vi "RunInference.vi"(4 "Introspection Output":T1, 6 "outputIndex":i32, 8 "error in (no error)":errorcluster, 9 "inputIndex":i32, 10 "inputBuffer":sgl[](array[numeric]), 11 "session id in":i32) -> (0 "error out":errorcluster, 1 "Dims":i64[](array[numeric]), 2 "outputBuffer":sgl[](array[numeric]), 3 "session id out":i32, 5 "RunInference":bool)   [LabVIEW 2017, in "libonnx_wrapper.lvlib"]
doc: "/**\n * @brief Выполнить инференс (предсказание) модели\n * \n * Основная функция для получения предсказания от модели. Принимает входные данные,\n * передаёт их в нейросеть и записывает результат в выходной буфер.\n * \n * @param sessionId [IN] ID сессии\n * @param inputIndex [IN] Индекс входа (обычно 0 для моделей с одним входом)\n * @param inputBuffer [IN] Массив входных данных (тип должен соответствовать GetInputType)\n * @param inputSize [IN] Количество элементов во входном массиве\n * @param outputIndex [IN] Индекс выхода (обычно 0 для моделей с одним выходом)\n * @param outputBuffer [OUT] Массив для записи результатов (должен быть выделен в LabVIEW)\n * @param outputSize [IN] Размер выходного буфера в элементах\n * \n * @return int32: 0 при успешном выполнении инференса\n * @return int32: -1 при ошибке (сессия не загружена, неверные индексы, ошибка ONNX Runtime)\n * \n * @note Входные данные должны быть нормализованы так же, как при обучении модели\n * @note Размер входного массива должен соответствовать произведению всех размерностей shape\n * @note Выходной буфер должен быть достаточного размера (см. GetOutputShapeDim)\n * @note Функция блокирует выполнение до завершения инференса\n * \n * @example\n * // Для модели с входом [1, 10] и выходом [1, 3]:\n * float inputData[10] = {...};\n * float outputData[3];\n * RunInference(sessionId, 0, inputData, 10, 0, outputData, 3);\n */\nint RunInference(int sessionId, int inputIndex, float* inputBuffer, int inputSize, \n int outputIndex, float* outputBuffer, int outputSize);"
uses:
  libonnx_wrapper.lvlib
  TypeDef/IO.ctl
  TypeDef/Introspection.ctl
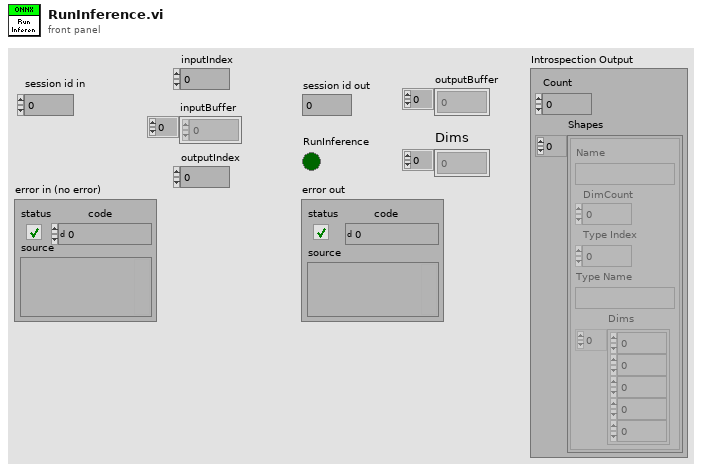
[diagram p1: front panel]
types:
  T1 = typedef "libonnx_wrapper.lvlib/Introspection.ctl" = cluster{"Count":i32, "Shapes":T2[]}
  T2 = typedef "libonnx_wrapper.lvlib/IO.ctl" = cluster{"Name":string, "DimCount":i32, "Type Index":i32, "Type Name":string, "Dims":i64[]}
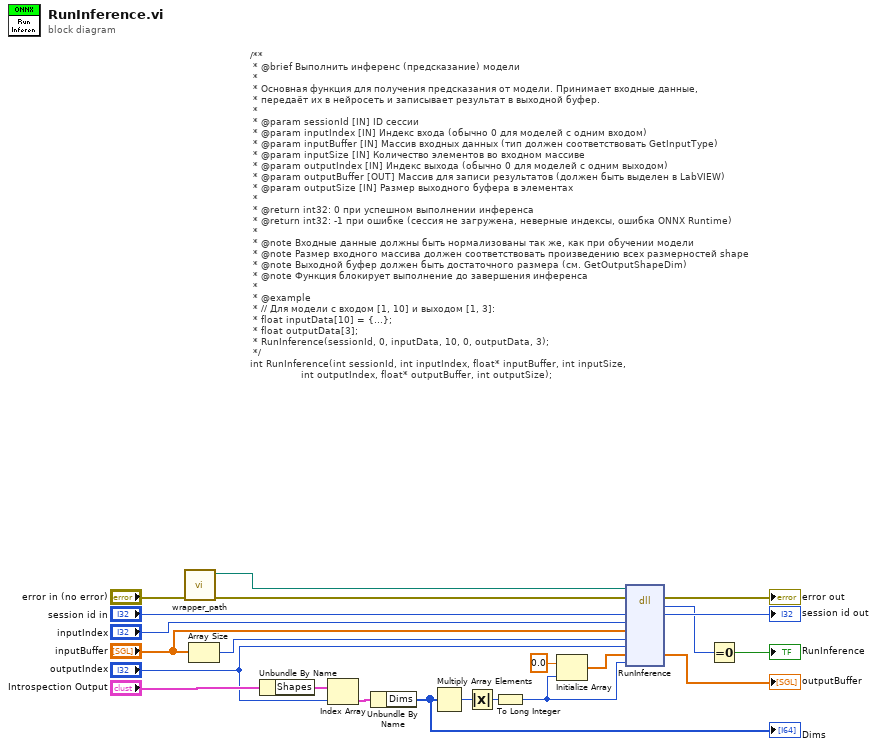
[diagram p0: block diagram]
diagram:
  # "/**\n * @brief Выполнить инференс (предсказание) модели\n * \n * Основная функция для получения предсказания от модели. Принимает входные данные,\n * передаёт их в нейросеть и записывает результат в выходной буфер.\n * \n * @param sessionId [IN] ID сессии\n * @param inputIndex [IN] Индекс входа (обычно 0 для моделей с одним входом)\n * @param inputBuffer [IN] Массив входных данных (тип должен соответствовать GetInputType)\n * @param inputSize [IN] Количество элементов во входном массиве\n * @param outputIndex [IN] Индекс выхода (обычно 0 для моделей с одним выходом)\n * @param outputBuffer [OUT] Массив для записи результатов (должен быть выделен в LabVIEW)\n * @param outputSize [IN] Размер выходного буфера в элементах\n * \n * @return int32: 0 при успешном выполнении инференса\n * @return int32: -1 при ошибке (сессия не загружена, неверные индексы, ошибка ONNX Runtime)\n * \n * @note Входные данные должны быть нормализованы так же, как при обучении модели\n * @note Размер входного массива должен соответствовать произведению всех размерностей shape\n * @note Выходной буфер должен быть достаточного размера (см. GetOutputShapeDim)\n * @note Функция блокирует выполнение до завершения инференса\n * \n * @example\n * // Для модели с входом [1, 10] и выходом [1, 3]:\n * float inputData[10] = {...};\n * float outputData[3];\n * RunInference(sessionId, 0, inputData, 10, 0, outputData, 3);\n */\nint RunInference(int sessionId, int inputIndex, float* inputBuffer, int inputSize, \n                 int outputIndex, float* outputBuffer, int outputSize);"
  n1 = call "wrapper_path.vi"("error in (no error)"="error in (no error)") -> ("error out"=w19:errorcluster, "wrapper path"=w20:path)  [unwired: 9 in]
  n2 = Array Size(array="inputBuffer") -> (size(s)=w12:i32)
  n3 = Unbundle By Name("Introspection Output") -> ("Shapes"=w8:T2[])
  n4 = Index Array(array=w8, index="outputIndex") -> (element=w7:T2)
  n5 = Unbundle By Name(w7) -> ("Dims"=w6:i64[])
  "Dims" <- w6
  n6 = Multiply Array Elements(1:w6) -> (0:w5:i64)
  n7 = Absolute Value(x=w5) -> (abs(x)=w4:i64)
  n8 = To Long Integer(number=w4) -> (32bit integer=w3:i32)
  n9 = Initialize Array(sgl 0.0 ("element"), w3) -> (w10:sgl[])
  n10 = dll-call lib="home/ivan/LabVIEWData/ONNX/Test/libonnx_wrapper/unix64/libonnx_wrapper.*" fn="RunInference"(path in=w20, error in=w19, "sessionId"="session id in", "inputIndex"="inputIndex", "inputBuffer"="inputBuffer", "inputSize"=w12, "outputIndex"="outputIndex", "outputBuffer"=w10, "outputSize"=w3) -> (error out=→"error out":errorcluster, "return type"=w15:i32, "sessionId"=→"session id out":i32, "outputBuffer"=→"outputBuffer":sgl[])  [unwired: 6 in, 1 out]
  n11 = Equal To 0?(x=w15) -> (x = 0?=→"RunInference":bool)
